vi "programa 6.vi"() -> ()   [LabVIEW 2011]
panel:
  out "Alarma":bool
  out "Temperatura":i32(slide) scale=0.0..100.0
  out "Cuarta":bool
  out "Tercera":bool
  out "Segunda":bool
  out "Primera":bool
  out "Velocidad":i32(knob) scale=0.0..180.0
  # "Deberá de generar la velocidad en número entero.\nLuego de acuerdo a la siguiente tabla:\n1-30 primera\n31-50 segunda\n51-85 tercera\n86-180 cuarta\nDeberá de encender las luces de los cambios.\n\nEncender la alarma cuando la temperatura sobrepase\nlos 80 grados y la velocidad es mayor a 150."
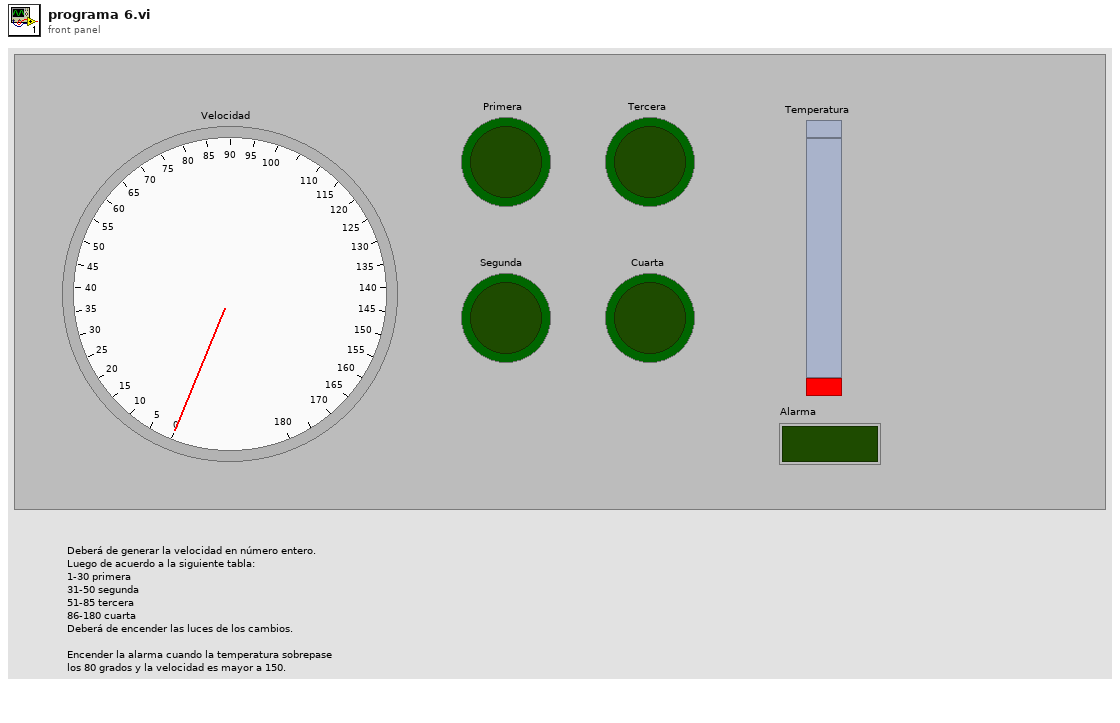
[diagram p1: front panel]
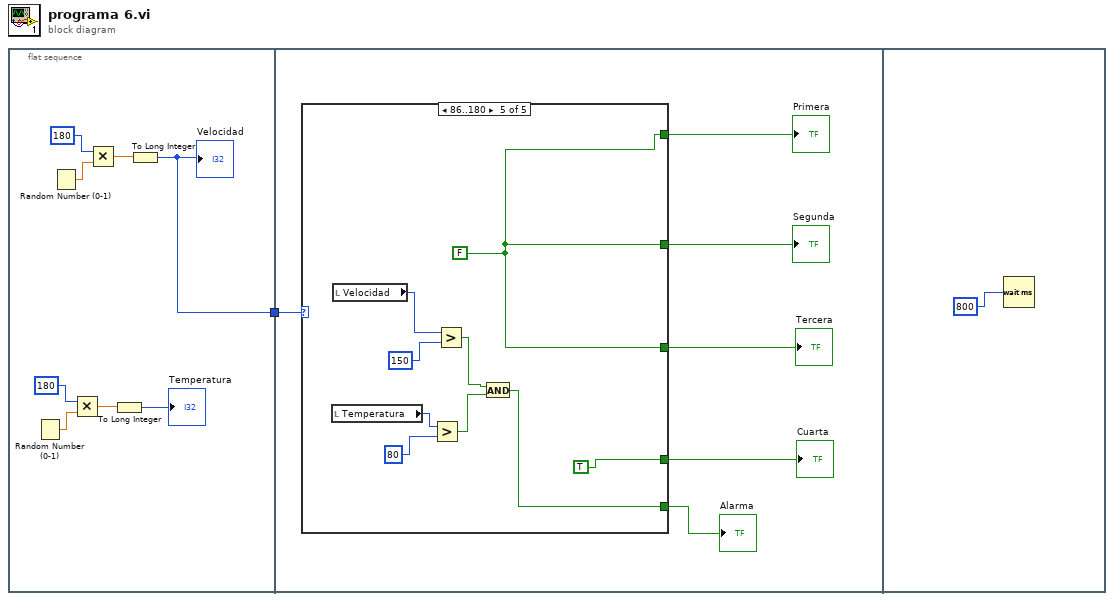
[diagram p0: block diagram]
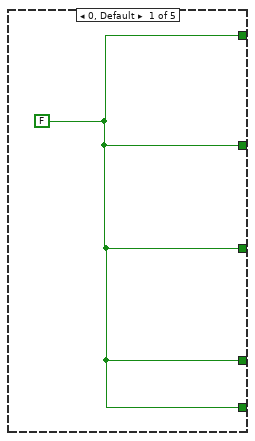
[diagram p2: hidden frame]
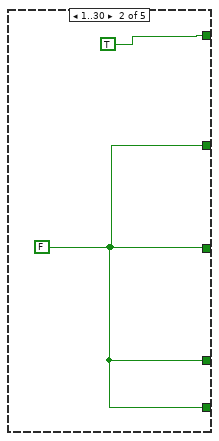
[diagram p3: hidden frame]
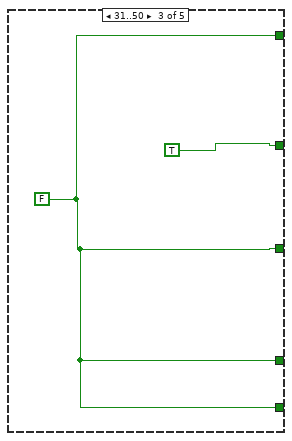
[diagram p4: hidden frame]
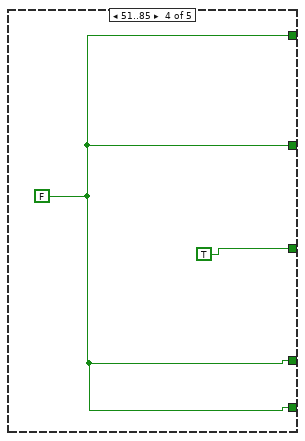
[diagram p5: hidden frame]
diagram:
  n1 = flat-sequence {
    tunnel: [w6] -> w1
    tunnel: w1 -> [w15]
    frame #0 {
      n2 = Random Number (0-1)() -> (number: 0 to 1=w4:dbl)
      n3 = Random Number (0-1)() -> (number: 0 to 1=w8:dbl)
      n4 = Multiply(x=180, y=w4) -> (x*y=w5:dbl)
      n5 = Multiply(x=180, y=w8) -> (x*y=w7:dbl)
      n6 = To Long Integer(number=w5) -> (32bit integer=→"Temperatura":i32)
      n7 = To Long Integer(number=w7) -> (32bit integer=w6:i32)
      "Velocidad" <- w6
    }
    frame #1 {
      n8 = case shown="86..180" w15 {
        tunnel: [w16 TRUE w19 w21 w30] -> w14
        tunnel: [w16 w17 TRUE w21 w30] -> w13
        tunnel: [w16 w17 w19 TRUE w30] -> w12
        tunnel: [w16 w17 w19 w21 TRUE] -> w11
        tunnel: [w16 w17 w19 w21 w23] -> w10
        frame 0, Default {
          w16 = FALSE
        }
        frame 1..30 {
          w17 = FALSE
        }
        frame 31..50 {
          w19 = FALSE
        }
        frame 51..85 {
          w21 = FALSE
        }
        frame 86..180 {
          w30 = FALSE
          n9 = local read "Temperatura"() -> (w26:i32)
          n10 = local read "Velocidad"() -> (w29:i32)
          n11 = Greater?(x=w26, y=80) -> (0:w24:bool)
          n12 = Greater?(x=w29, y=150) -> (0:w25:bool)
          n13 = And(x=w25, y=w24) -> (x .and. y?=w23:bool)
        }
      }
      "Primera" <- w14
      "Segunda" <- w13
      "Tercera" <- w12
      "Cuarta" <- w11
      "Alarma" <- w10
    }
    frame #2 {
      n14 = Wait (ms)(milliseconds to wait=800) -> ()  [unwired: 1 out]
    }
  }
